vi "DlgConfirmCalcSummary_TempTest.vi"(8 "error in (no error)":errorcluster, 10 "Path":path, 11 "PMUConfig 2":T1={"Class"="", "Fs"=0.0, "F0"=0.0, "Temp"="50C"}) -> (0 "error out":errorcluster, 1 "Summary Data Excel File":path, 2 "Path":path, 3 "PMUConfig":T1={"Class"="", "Fs"=0.0, "F0"=0.0, "Temp"="50C"})   [LabVIEW 2014]
uses:
  typedef/PMUConfig_TempTests.ctl
  typedef/appState.ctl
panel:
  in  "BtnAbort":bool
  in  "BtnSkip":bool
  in  "BtnChange":bool
  in  "BtnProcess":bool
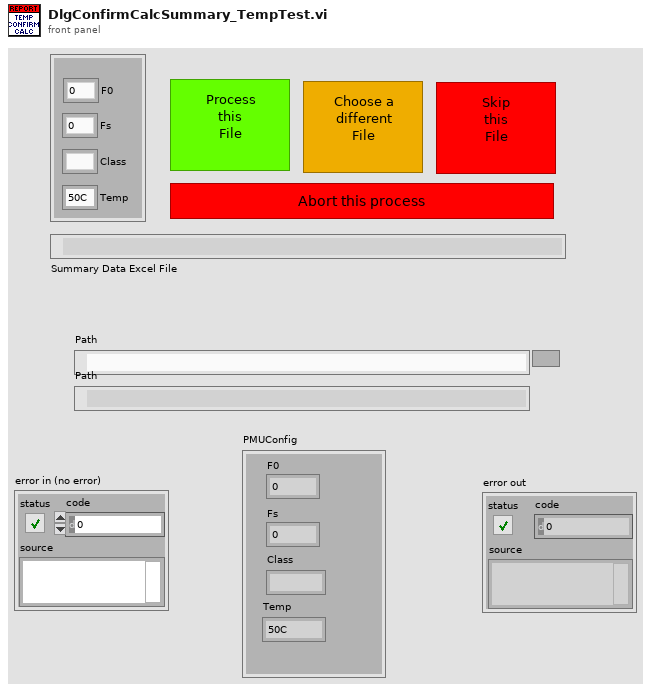
[diagram p1: front panel]
types:
  T1 = typedef "PMUConfig_TempTests.ctl" = cluster{"Class":string, "Fs":dbl, "F0":dbl, "Temp":string}
  T2 = typedef "appState.ctl" = enum16{"init", "processUI", "exit"}
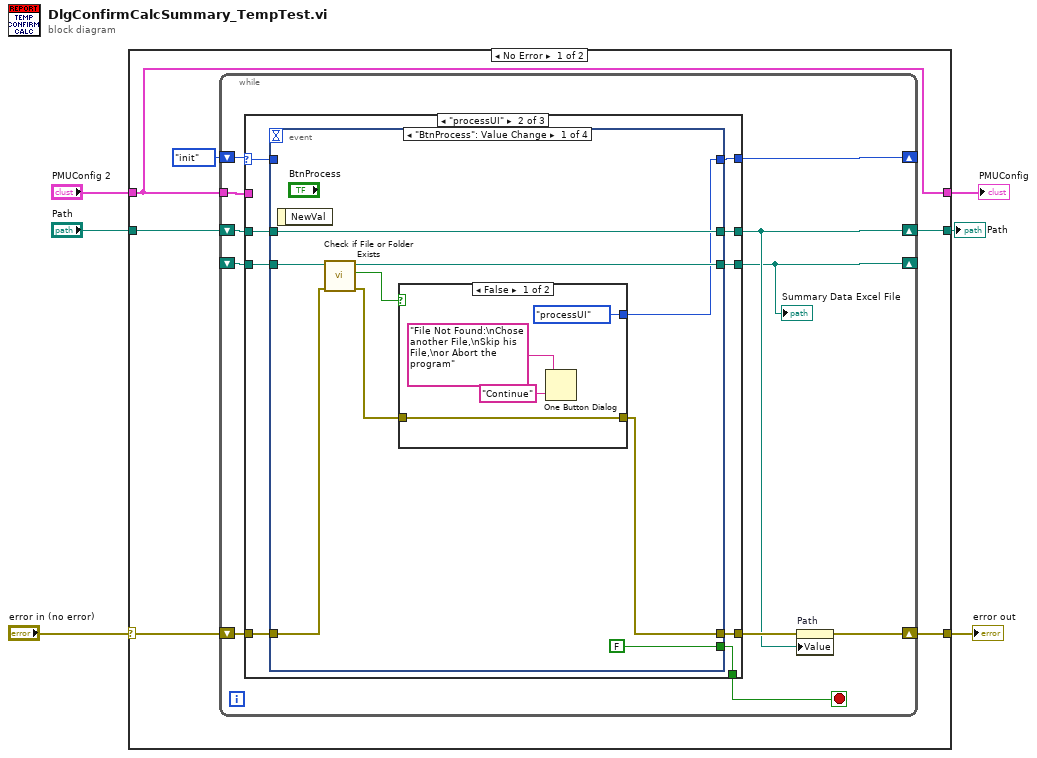
[diagram p0: block diagram]
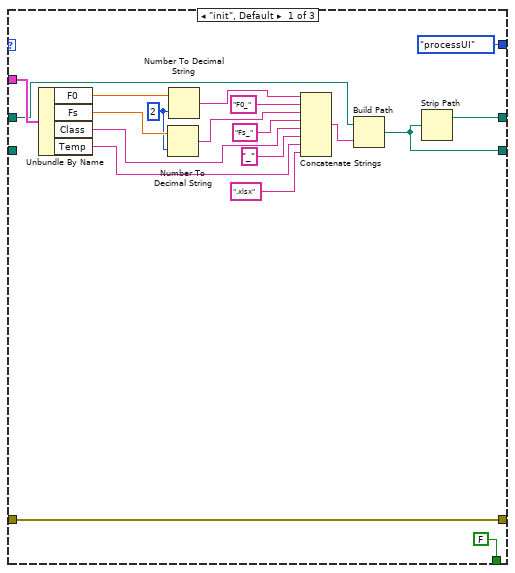
[diagram p2: hidden frame]
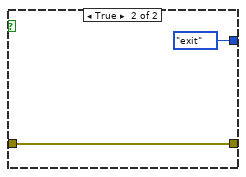
[diagram p3: hidden frame]
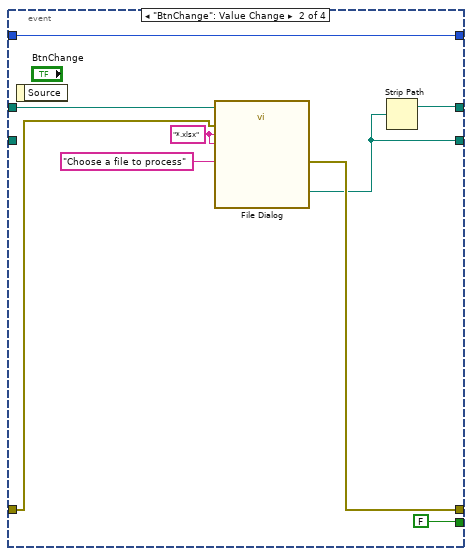
[diagram p4: hidden frame]
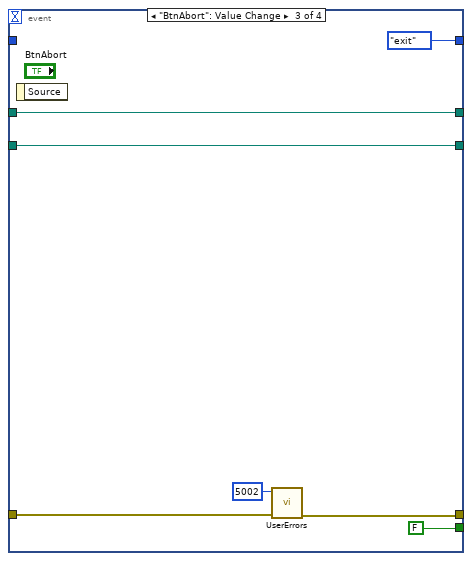
[diagram p5: hidden frame]
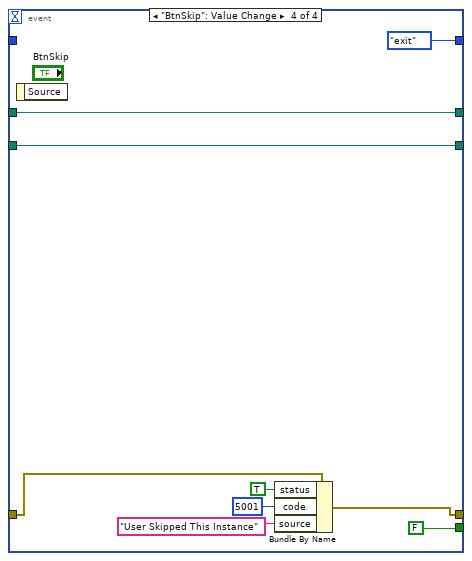
[diagram p6: hidden frame]
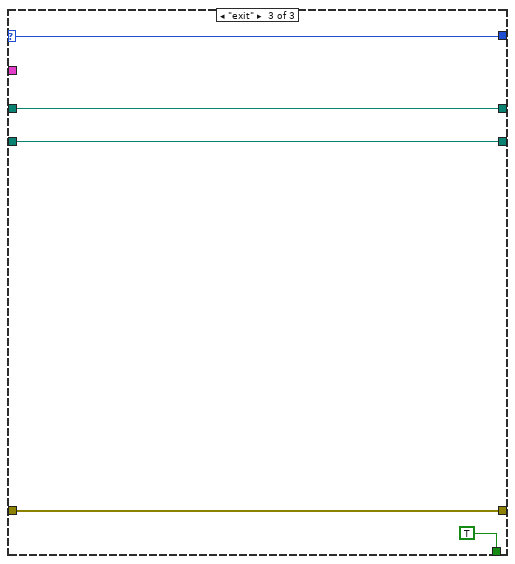
[diagram p7: hidden frame]
diagram:
  n1 = case shown="No Error" "error in (no error)" {
    selector: "error in (no error)" -> [w10 w99]
    tunnel: [w9 w99] -> w5
    tunnel: "PMUConfig 2" -> [w7 w97]
    tunnel: "Path" -> [w11 w98]
    tunnel: [w8 w98] -> w2
    tunnel: [w7 w97] -> w1
    frame No Error {
      n2 = while {
        tunnel: w7 -> [w22]
        shift-right: [w15] -> w9
        shift-left: w10 -> [w20]
        shift-right: [w17] -> _
        shift-left: appState."init" ("AppState") -> [w23]
        shift-right: [w14] -> w8
        shift-left: w11 -> [w21]
        shift-right: [w13] -> _
        shift-left: _ -> [w18]
        stop <- w19 stop-if-true
        n3 = case shown="\"processUI\"" w23 {
          selector: w23 -> [_ w50 w96]
          tunnel: w22 -> [w41 _ _]
          tunnel: w21 -> [w32 w48 w94]
          tunnel: w20 -> [w42 w44 w92]
          tunnel: [w42 w43 w92] -> w16
          tunnel: [w29 w45 w93] -> w13
          tunnel: [FALSE w51 TRUE] -> w19
          tunnel: [w28 w47 w94] -> w14
          tunnel: w18 -> [_ w46 w93]
          tunnel: [appState."processUI" ("AppState") w49 w96] -> w17
          frame "init", Default {
            w37 = i16 2 ("width (-)")
            n4 = Unbundle By Name(w41) -> ("F0"=w39:dbl, "Fs"=w38:dbl, "Class"=w27:string, "Temp"=w25:string)
            n5 = Number To Decimal String(number=w38, width (-)=w37) -> (decimal integer string=w33:string)
            n6 = Number To Decimal String(number=w39, width (-)=w37) -> (decimal integer string=w34:string)
            n7 = Concatenate Strings(w34, "F0_" ("string"), w33, "Fs_" ("string"), w27, "_" ("string"), w25, ".xlsx" ("string")) -> (w31:string)
            n8 = Build Path(base path=w32, name or relative path=w31) -> (appended path=w29:path)
            n9 = Strip Path(path=w29) -> (stripped path=w28:path)  [unwired: 1 out]
          }
          frame "processUI" {
            n10 = event shown="[0] \"BtnProcess\": Value Change" {
              selector: _ -> [_ _ _ _]
              dyn-events: _ -> [_ _ _ _]
              timeout: _ -> [_ _ _ _]
              tunnel: [FALSE FALSE FALSE FALSE] -> w51
              tunnel: w50 -> [_ w75 _ _]
              tunnel: [w52 w75 appState."exit" ("AppState") appState."exit" ("AppState")] -> w49
              tunnel: w48 -> [w59 w74 w78 w90]
              tunnel: [w59 w67 w78 w90] -> w47
              tunnel: [w57 w68 w77 w89] -> w45
              tunnel: w46 -> [w58 _ w77 w89]
              tunnel: w44 -> [w54 w71 w80 w83]
              tunnel: [w53 w70 w79 w84] -> w43
              event "BtnProcess": Value Change {
                n11 = event-data() -> ()  [unwired: 1 in, 1 out]
                n12 = call <vilib>:"Check if File or Folder Exists.vi"("error in (no error)"=w54, "path"=w58) -> ("error out"=w55:errorcluster, "file or folder exists?"=w56:bool, "dup path"=w57:path)  [unwired: 7 in]
                n13 = case shown="False" w56 {
                  tunnel: w55 -> [w62 w66]
                  tunnel: [w62 w66] -> w53
                  tunnel: [appState."processUI" ("AppState") appState."exit" ("AppState")] -> w52
                  frame False {
                    n14 = One Button Dialog(message="File Not Found:\nChose another File,\nSkip his File,\nor Abort the program", button name ("OK")="Continue") -> ()  [unwired: 1 out]
                  }
                  frame True {
                  }
                }
              }
              event "BtnChange": Value Change {
                w73 = "*.xlsx" ("pattern (all files)")
                n15 = event-data() -> ()  [unwired: 1 in, 1 out]
                n16 = call "File Dialog"("start path"=w74, "prompt"="Choose a file to process", "error in"=w71, "pattern (all files)"=w73, "pattern label"=w73) -> ("selected path"=w68:path, "error out"=w70:errorcluster)  [unwired: 7 in, 2 out]
                n17 = Strip Path(path=w68) -> (stripped path=w67:path)  [unwired: 1 out]
              }
              event "BtnAbort": Value Change {
                n18 = event-data() -> ()  [unwired: 1 in, 1 out]
                n19 = call "UserErrors.vi"("error in (no error)"=w80, "[error code] (0)"=5002) -> ("error out"=w79:errorcluster)  [unwired: 9 in]
              }
              event "BtnSkip": Value Change {
                n20 = event-data() -> ()  [unwired: 1 in, 1 out]
                n21 = Bundle By Name(cluster=w83, "status"=TRUE, "code"=5001 ("[error code] (0)"), "source"="User Skipped This Instance") -> (w84:errorcluster)
              }
            }
          }
          frame "exit" {
          }
        }
        "Summary Data Excel File" <- w13
        n22 = property on="Path" class="Path"(error in=w16, "Value"=w14) -> (error out=w15:errorcluster)  [unwired: 1 in, 1 out]
      }
    }
    frame Error {
    }
  }
  "PMUConfig" <- w1
  "error out" <- w5
  "Path" <- w2
